vi "4Pi Capture File Name Increment.vi"(0 "Path In":path, 5 "Laser Line":string, 7 "Cycle":u16, 9 "Step":u16, 11 "Mirror Mode":u16, 12 "Amp step":u16, 13 "add DM":bool) -> (4 "Path Out":path)   [LabVIEW 2021]
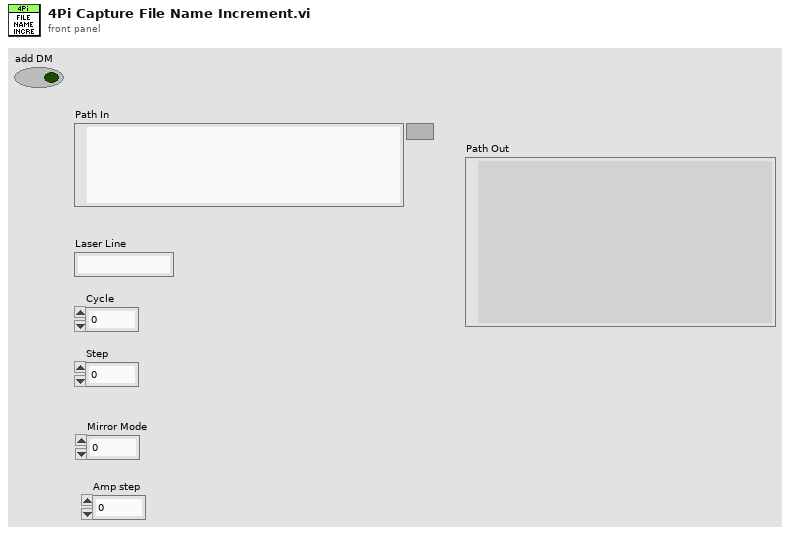
[diagram p1: front panel]
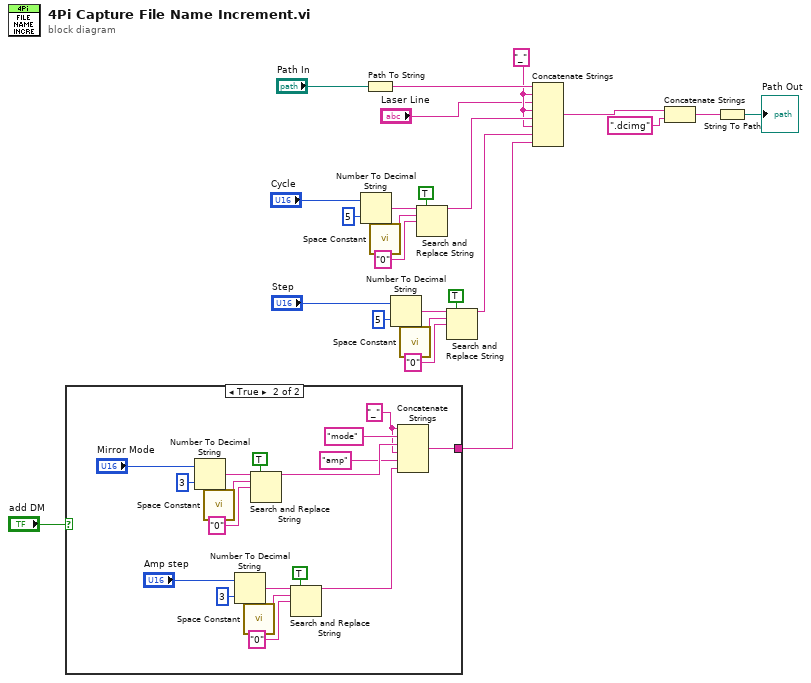
[diagram p0: block diagram]
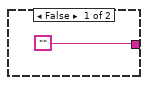
[diagram p2: hidden frame]
diagram:
  w12 = "_" ("string")
  n1 = case shown="True" "add DM" {
    tunnel: ["" w26] -> w1
    frame False {
    }
    frame True {
      w35 = "_" ("string")
      n2 = Number To Decimal String(number="Mirror Mode", width (-)=i16 3) -> (decimal integer string=w40:string)
      n3 = call <vilib>:"Space Constant.vi"() -> ("String"=w41:string)
      n4 = Number To Decimal String(number="Amp step", width (-)=i16 3) -> (decimal integer string=w30:string)
      n5 = call <vilib>:"Space Constant.vi"() -> ("String"=w31:string)
      n6 = Search and Replace String(replace all?=TRUE ("replace all? (F)"), input string=w40, search string=w41, replace string="0" ("replace string (\"\")")) -> (result string=w36:string)  [unwired: 4 in, 3 out]
      n7 = Search and Replace String(replace all?=TRUE ("replace all? (F)"), input string=w30, search string=w31, replace string="0" ("replace string (\"\")")) -> (result string=w27:string)  [unwired: 4 in, 3 out]
      n8 = Concatenate Strings(w35, "mode" ("string"), w36, w35, "amp" ("string"), w27) -> (w26:string)
    }
  }
  n9 = Number To Decimal String(number="Cycle", width (-)=i16 5) -> (decimal integer string=w20:string)
  n10 = Path To String(path="Path In") -> (string=w24:string)
  n11 = call <vilib>:"Space Constant.vi"() -> ("String"=w21:string)
  n12 = Number To Decimal String(number="Step", width (-)=i16 5) -> (decimal integer string=w17:string)
  n13 = call <vilib>:"Space Constant.vi"() -> ("String"=w16:string)
  n14 = Search and Replace String(replace all?=TRUE ("replace all? (F)"), input string=w20, search string=w21, replace string="0" ("replace string (\"\")")) -> (result string=w13:string)  [unwired: 4 in, 3 out]
  n15 = Search and Replace String(replace all?=TRUE ("replace all? (F)"), input string=w17, search string=w16, replace string="0" ("replace string (\"\")")) -> (result string=w11:string)  [unwired: 4 in, 3 out]
  n16 = Concatenate Strings(w24, w12, "Laser Line", w12, w13, w12, w11, w1) -> (w10:string)
  n17 = Concatenate Strings(w10, ".dcimg" ("string")) -> (w9:string)
  n18 = String To Path(string=w9) -> (path=→"Path Out":path)
